vi "Config Mapping.vi"(8 "error in (no error)":errorcluster, 11 "HW InOut MAP in":T2) -> (0 "error out":errorcluster, 3 "HW InOut MAP out":T2)   [LabVIEW 2014, in "SeqLoop.lvlib"]
doc: "Configura el mapeo de entradas y salidas digitales."
uses:
  TypeDefs/HW InOut MAP.ctl
  SeqLoop.lvlib
panel:
  out "Array":T1(array[cluster])
  in  "IO Config":T3(tab)
  in  "Edit Map In":bool
  in  "I Config":i32(listbox)=-1 caption="Secuencia"
  in  "Add Map In":bool
  in  "Delete Map In":bool
  in  "Stop Map In":bool
  in  "Edit Map Out":bool
  in  "Out Config":i32(listbox)=-1 caption="Secuencia"
  in  "Add Map Out":bool
  in  "Delete Map Out":bool
  in  "Stop Map Out":bool
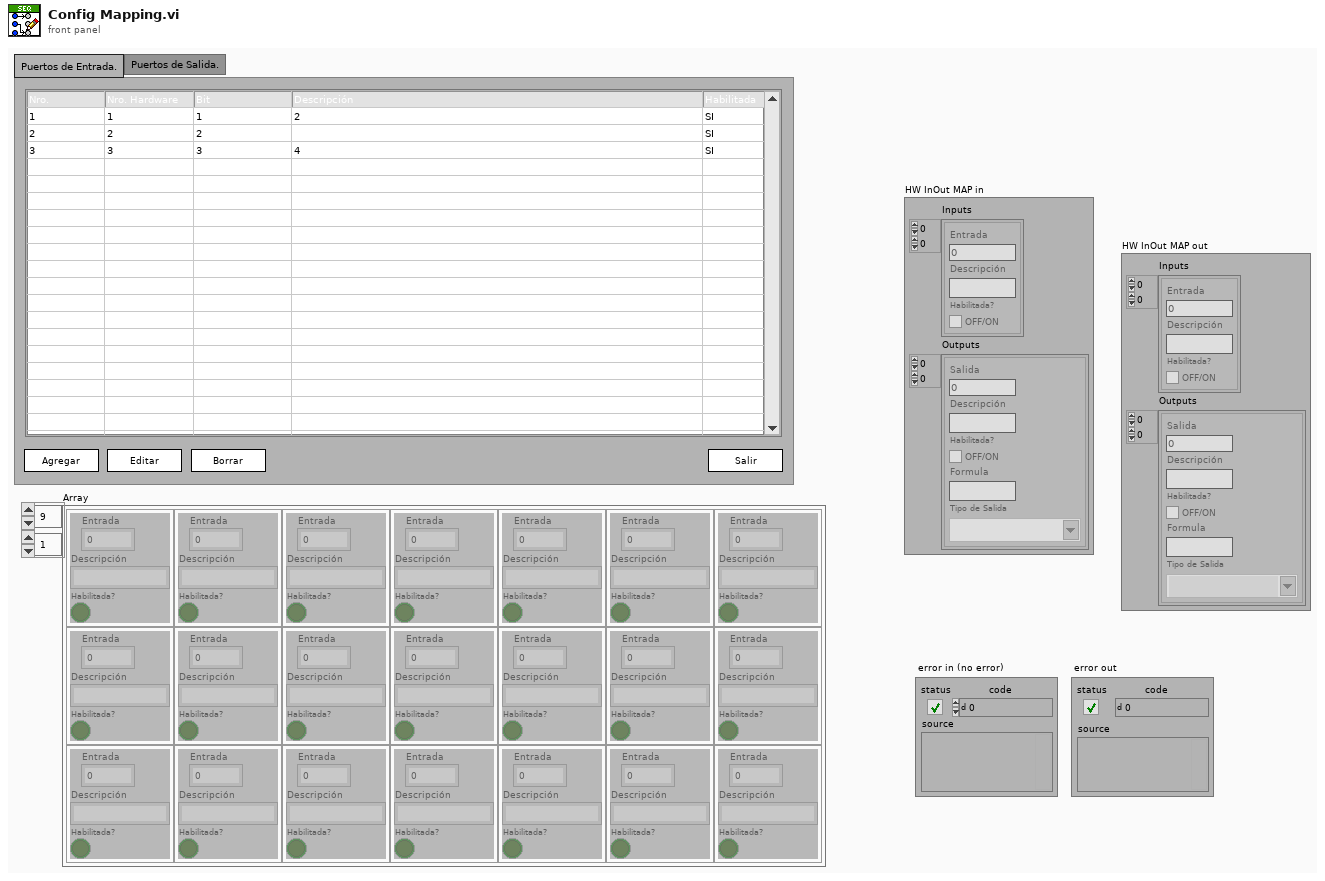
[diagram p1: front panel]
types:
  T1 = cluster{"Entrada":i32, "Descripción":string, "Habilitada?":bool}[][]
  T2 = typedef "SeqLoop.lvlib/HW InOut MAP.ctl" = cluster{"Inputs":cluster{"Entrada":i32, "Descripción":string, "Habilitada?":bool}[][], "Outputs":cluster{"Salida":i32, "Descripción":string, "Habilitada?":bool, "Formula":string, "Tipo de Salida":string}[][]}
  T3 = enum32{"Puertos de Entrada.", "Puertos de Salida."}
  T4 = cluster{"Entrada":i32, "Descripción":string, "Habilitada?":bool, "Formula":string, "Tipo de Salida":string}
  T5 = cluster{"Entrada":i32, "Descripción":string, "Habilitada?":bool}
  T6 = enum8{"Enabled", "Disabled", "Disabled and Grayed Out"}
  T7 = cluster{"Salida":i32, "Descripción":string, "Habilitada?":bool, "Formula":string, "Tipo de Salida":string}[][]
  T8 = cluster{"Entrada":i32, "Descripción":string, "Habilitada?":bool, "Formula":string, "Tipo de Salida":string}[][]
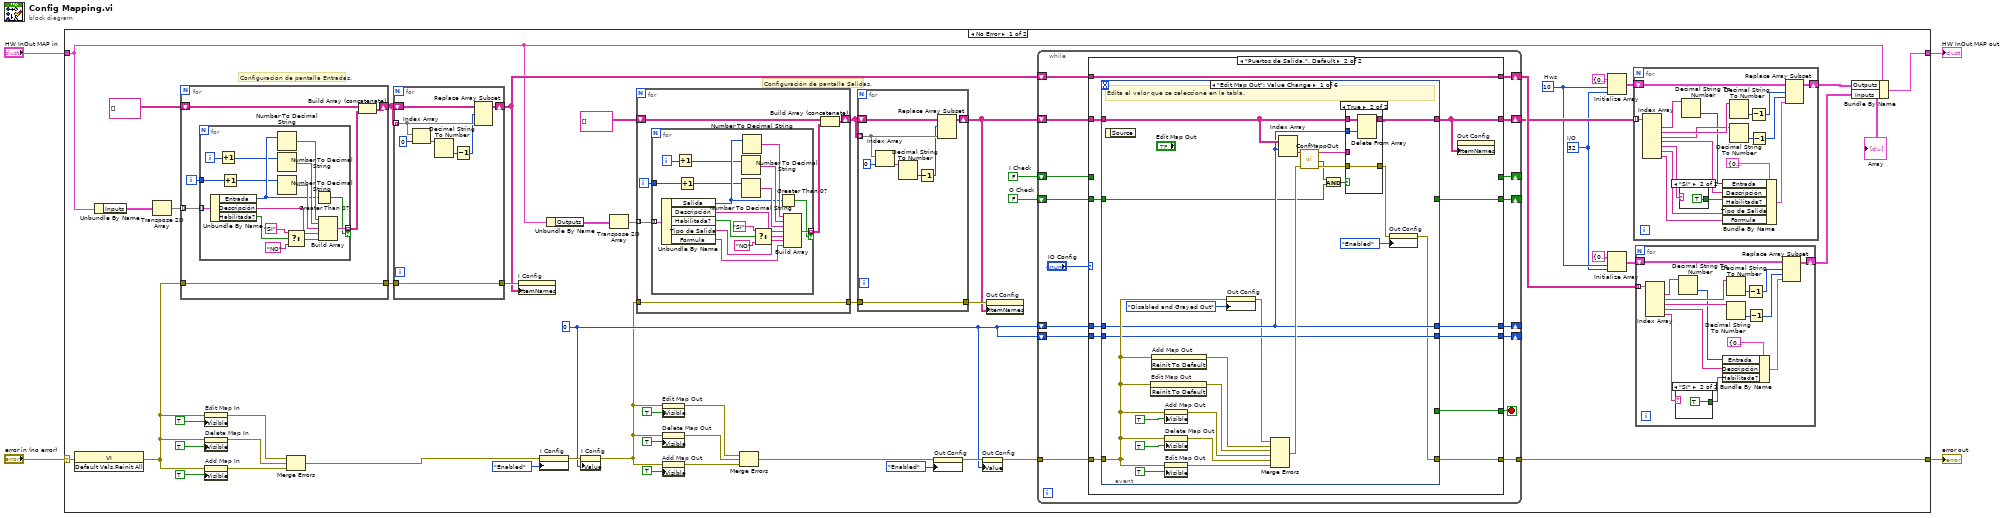
[diagram p0: block diagram]
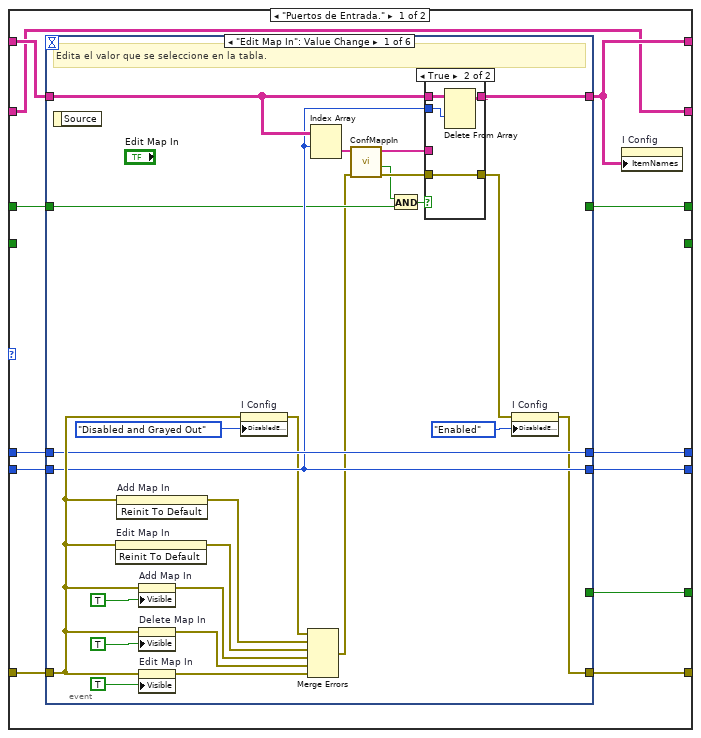
[diagram p4: hidden frame]
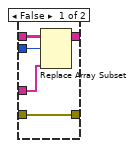
[diagram p5: hidden frame]
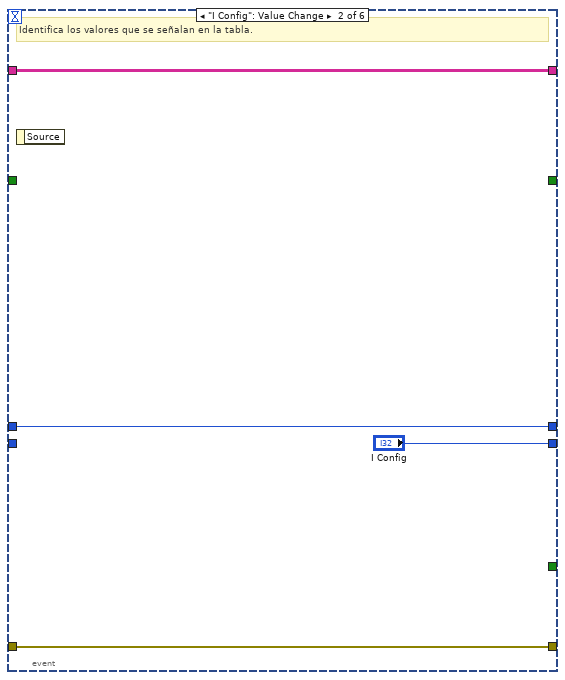
[diagram p6: hidden frame]
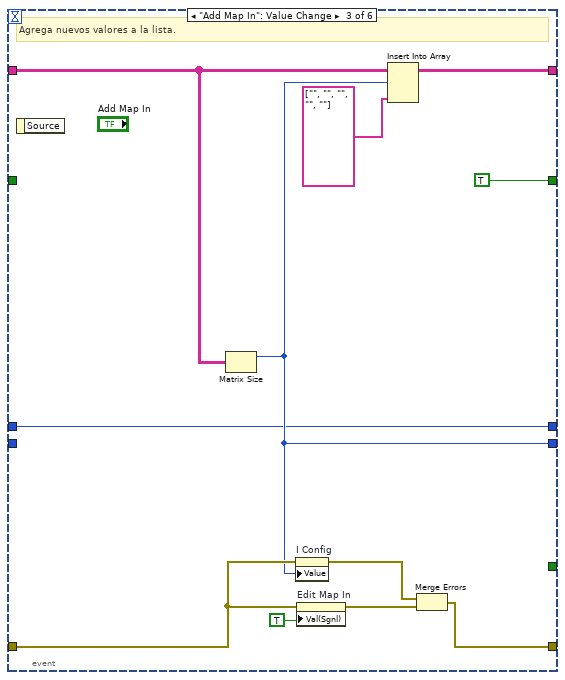
[diagram p7: hidden frame]
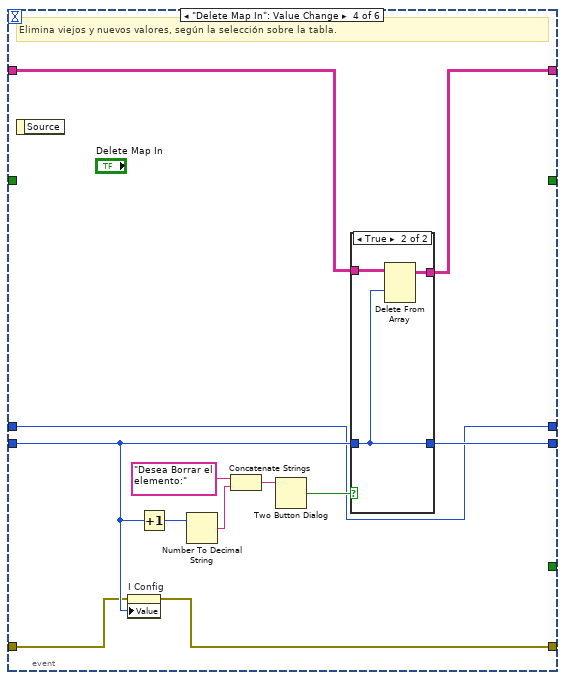
[diagram p8: hidden frame]
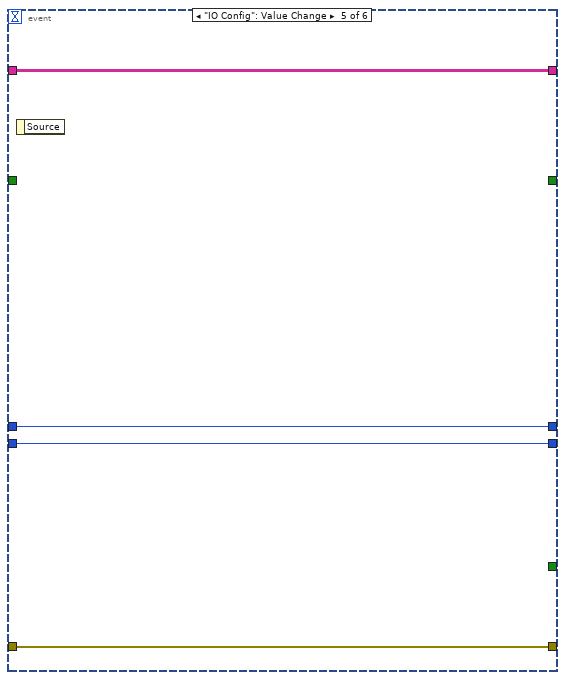
[diagram p10: hidden frame]
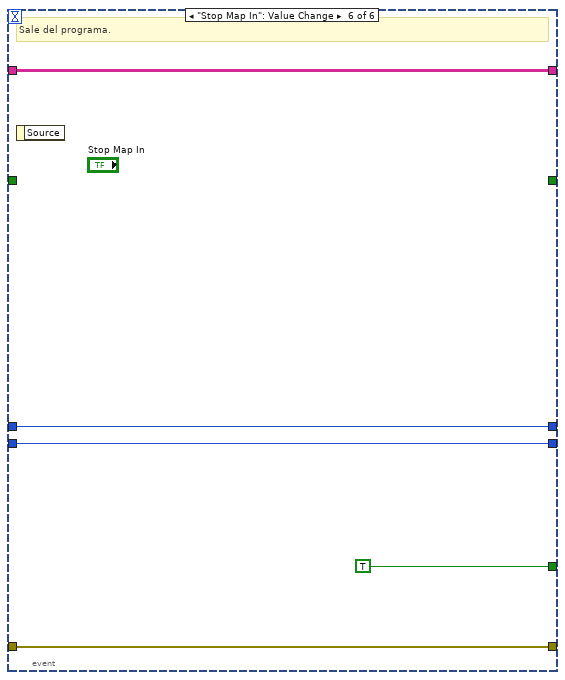
[diagram p11: hidden frame]
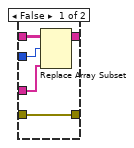
[diagram p12: hidden frame]
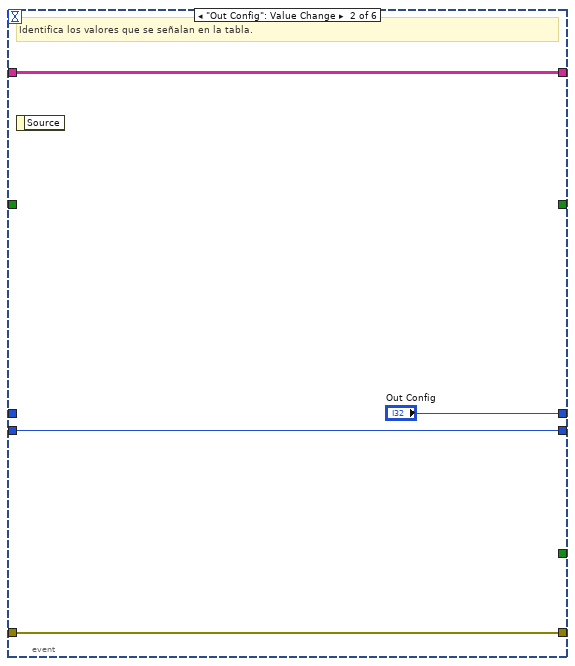
[diagram p13: hidden frame]
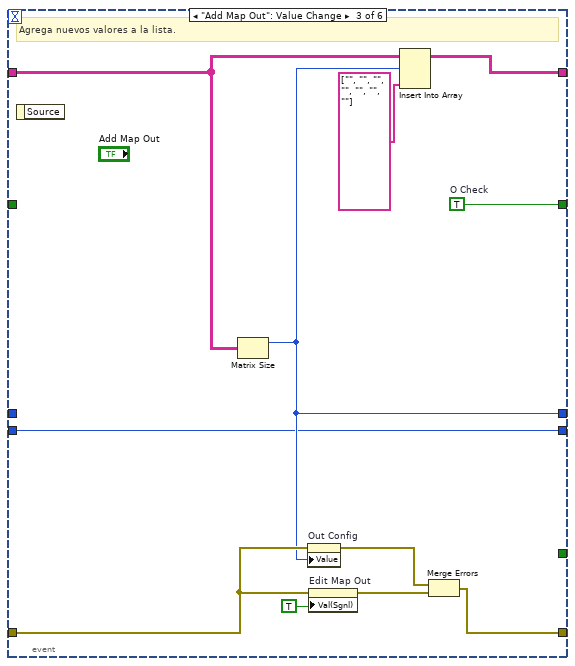
[diagram p14: hidden frame]
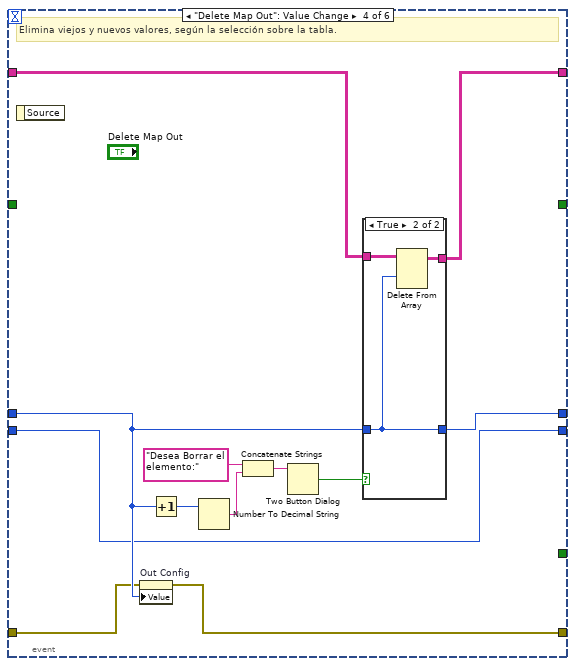
[diagram p15: hidden frame]
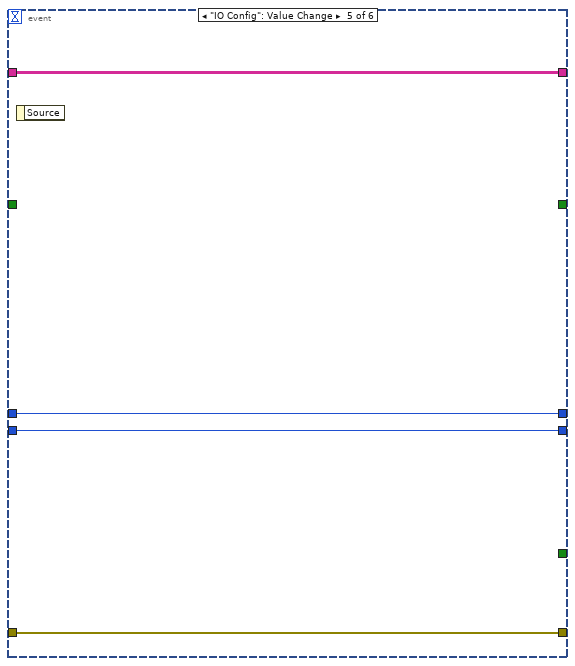
[diagram p17: hidden frame]
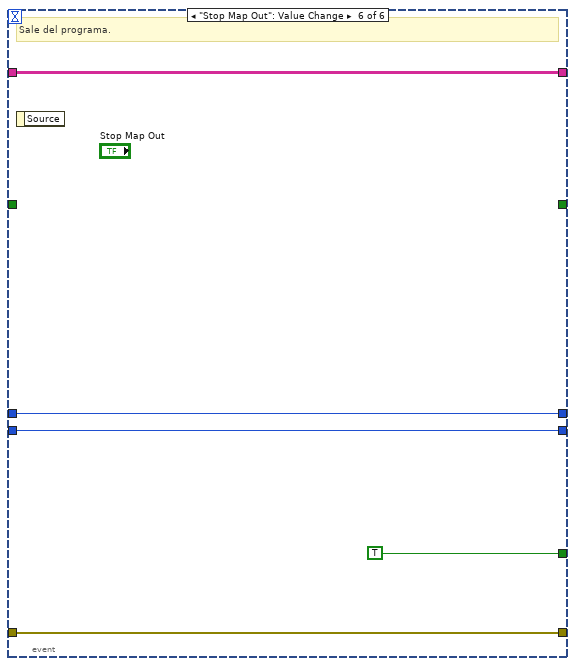
[diagram p18: hidden frame]
diagram:
  n1 = case shown="No Error" "error in (no error)" {
    selector: "error in (no error)" -> [w55 w346]
    tunnel: [w56 w346] -> w4
    tunnel: "HW InOut MAP in" -> [w19 w345]
    tunnel: [w34 w345] -> w1
    frame No Error {
      w5 = FALSE  # O Check
      w6 = FALSE  # I Check
      w11 = 32  # I/O
      w12 = 10  # Hws
      w36 = 0 ("disabled index (col)")
      # "Configuración de pantalla Entradas."
      # "Configuración de pantalla Salidas."
      n2 = invoke class="VI" method="Default Vals.Reinit All"(error in=w55) -> (error out=w22:errorcluster)  [unwired: 2 in, 2 out]
      n3 = Unbundle By Name(w19) -> ("Inputs"=w10:T1)
      n4 = Transpose 2D Array(2D array=w10) -> (transposed array=w9:T1)
      n5 = for {
        tunnel: w9 -> [w87] mode=indexing
        shift-right: [w83] -> w24
        shift-left: string[][] [] -> [w85]
        tunnel: w22 -> [w82]
        tunnel: [w82] -> w26
        i -> [w86]
        n6 = for {
          tunnel: w87 -> [w103] mode=indexing
          tunnel: w86 -> [w91]
          tunnel: [w98] -> w84 mode=indexing if=w92
          i -> [w89]
          n7 = Unbundle By Name(w103) -> ("Entrada"=w93:i32, "Descripción"=w94:string, "Habilitada?"=w102:bool)
          n8 = Increment(x=w89) -> (x+1=w88:i32)
          n9 = Increment(x=w91) -> (x+1=w90:i32)
          n10 = Number To Decimal String(number=w88) -> (decimal integer string=w97:string)  [unwired: 1 in]
          n11 = Number To Decimal String(number=w90) -> (decimal integer string=w96:string)  [unwired: 1 in]
          n12 = Number To Decimal String(number=w93) -> (decimal integer string=w99:string)  [unwired: 1 in]
          n13 = Select(t="SI" ("Descripción"), s=w102, f="NO" ("Descripción")) -> (s? t:f=w95:string)
          n14 = Greater Than 0?(x=w93) -> (x > 0?=w92:bool)
          n15 = Build Array(w99, w97, w96, w94, w95) -> (w98:string[])
        }
        n16 = Build Array (concatenate)(w85, w84) -> (w83:string[][])
      }
      n17 = property on="Edit Map In" class="Bool (strict)"(error in=w22, "Visible"=TRUE) -> (error out=w47:errorcluster)  [unwired: 1 in, 1 out]
      n18 = property on="Delete Map In" class="Bool"(error in=w22, "Visible"=TRUE) -> (error out=w49:errorcluster)  [unwired: 1 in, 1 out]
      n19 = property on="Add Map In" class="Bool (strict)"(error in=w22, "Visible"=TRUE) -> (error out=w51:errorcluster)  [unwired: 1 in, 1 out]
      n20 = Merge Errors(w47, w49, w51) -> (w53:errorcluster)
      n21 = for {
        tunnel: w24 -> [w79] mode=indexing
        shift-right: [w78] -> w21
        shift-left: w24 -> [w80]
        tunnel: [w74] -> w25
        tunnel: w26 -> [w74]
        n22 = Index Array(array=w79, index=0) -> (element=w77:string)
        n23 = Decimal String To Number(string=w77) -> (number=w76:i32)  [unwired: 2 in, 1 out]
        n24 = Decrement(x=w76) -> (x-1=w75:i32)
        n25 = Replace Array Subset(array=w80, new element=w79, index (row)=w75) -> (w78:string[][])  [unwired: 1 in]
      }
      n26 = property on="I Config" class="MCListbox (strict)"(error in=w25, "ItemNames"=w21) -> ()  [unwired: 1 in, 2 out]
      n27 = property on="I Config" class="MCListbox (strict)"(error in=w53, "DisabledEnum"=T6."Enabled" ("Disabled")) -> (error out=w54:errorcluster)  [unwired: 1 in, 1 out]
      n28 = Unbundle By Name(w19) -> ("Outputs"=w8:T7)
      n29 = property on="I Config" class="MCListbox (strict)"(error in=w54, "Value"=w36) -> (error out=w27:errorcluster)  [unwired: 1 in, 1 out]
      n30 = Transpose 2D Array(2D array=w8) -> (transposed array=w7:T7)
      n31 = for {
        tunnel: w7 -> [w117] mode=indexing
        shift-right: [w113] -> w30
        shift-left: string[][] [] -> [w115]
        tunnel: w27 -> [w112]
        tunnel: [w112] -> w32
        i -> [w116]
        n32 = for {
          tunnel: w117 -> [w135] mode=indexing
          tunnel: w116 -> [w123]
          tunnel: [w130] -> w114 mode=indexing if=w124
          i -> [w121]
          n33 = Unbundle By Name(w135) -> ("Salida"=w125:i32, "Descripción"=w126:string, "Habilitada?"=w134:bool, "Tipo de Salida"=w119:string, "Formula"=w118:string)
          n34 = Increment(x=w121) -> (x+1=w120:i32)
          n35 = Increment(x=w123) -> (x+1=w122:i32)
          n36 = Number To Decimal String(number=w120) -> (decimal integer string=w129:string)  [unwired: 1 in]
          n37 = Number To Decimal String(number=w122) -> (decimal integer string=w128:string)  [unwired: 1 in]
          n38 = Number To Decimal String(number=w125) -> (decimal integer string=w131:string)  [unwired: 1 in]
          n39 = Select(t="SI" ("Descripción"), s=w134, f="NO" ("Descripción")) -> (s? t:f=w127:string)
          n40 = Greater Than 0?(x=w125) -> (x > 0?=w124:bool)
          n41 = Build Array(w131, w129, w128, w126, w127, w119, w118) -> (w130:string[])
        }
        n42 = Build Array (concatenate)(w115, w114) -> (w113:string[][])
      }
      n43 = property on="Edit Map Out" class="Bool (strict)"(error in=w27, "Visible"=TRUE) -> (error out=w38:errorcluster)  [unwired: 1 in, 1 out]
      n44 = property on="Delete Map Out" class="Bool"(error in=w27, "Visible"=TRUE) -> (error out=w40:errorcluster)  [unwired: 1 in, 1 out]
      n45 = property on="Add Map Out" class="Bool (strict)"(error in=w27, "Visible"=TRUE) -> (error out=w42:errorcluster)  [unwired: 1 in, 1 out]
      n46 = Merge Errors(w38, w40, w42) -> (w44:errorcluster)
      n47 = for {
        tunnel: w30 -> [w109] mode=indexing
        shift-right: [w108] -> w28
        shift-left: w30 -> [w110]
        tunnel: [w104] -> w31
        tunnel: w32 -> [w104]
        n48 = Index Array(array=w109, index=0) -> (element=w107:string)
        n49 = Decimal String To Number(string=w107) -> (number=w106:i32)  [unwired: 2 in, 1 out]
        n50 = Decrement(x=w106) -> (x-1=w105:i32)
        n51 = Replace Array Subset(array=w110, new element=w109, index (row)=w105) -> (w108:string[][])  [unwired: 1 in]
      }
      n52 = property on="Out Config" class="MCListbox (strict)"(error in=w44, "DisabledEnum"=T6."Enabled" ("Disabled")) -> (error out=w45:errorcluster)  [unwired: 1 in, 1 out]
      n53 = property on="Out Config" class="MCListbox (strict)"(error in=w45, "Value"=w36) -> (error out=w33:errorcluster)  [unwired: 1 in, 1 out]
      n54 = property on="Out Config" class="MCListbox (strict)"(error in=w31, "ItemNames"=w28) -> ()  [unwired: 1 in, 2 out]
      n55 = while {
        tunnel: w33 -> [w169]
        tunnel: [w170] -> w56
        shift-right: [w166] -> _
        shift-left: w36 -> [w165]
        shift-right: [w164] -> _
        shift-left: w36 -> [w163]
        shift-right: [w162] -> w14
        shift-left: w28 -> [w161]
        shift-right: [w159] -> w17
        shift-left: w21 -> [w160]
        shift-right: [w157] -> _
        shift-left: w6 -> [w158]
        shift-right: [w155] -> _
        shift-left: w5 -> [w156]
        stop <- w167 stop-if-true
        n56 = case shown="\"Puertos de Salida.\", Default" "IO Config" {
          tunnel: [w182 w269] -> w170
          tunnel: w169 -> [w179 w264]
          tunnel: [w181 w268] -> w167
          tunnel: w165 -> [w176 w265]
          tunnel: [w180 w266] -> w166
          tunnel: [w178 w267] -> w164
          tunnel: w163 -> [w177 w263]
          tunnel: [w173 w262] -> w162
          tunnel: w161 -> [w173 w261]
          tunnel: w160 -> [w175 w260]
          tunnel: [w174 w260] -> w159
          tunnel: w158 -> [w172 _]
          tunnel: [w171 _] -> w157
          tunnel: w156 -> [_ w259]
          tunnel: [_ w258] -> w155
          frame "Puertos de Entrada." {
            n57 = event shown="[0] \"Edit Map In\": Value Change" {
              selector: _ -> [_ _ _ _ _ _]
              dyn-events: _ -> [_ _ _ _ _ _]
              timeout: _ -> [_ _ _ _ _ _]
              tunnel: w175 -> [w198 w220 w225 w241 w252 w256]
              tunnel: [w196 w220 w227 w240 w252 w256] -> w174
              tunnel: [w197 "I Config" w224 w242 w251 w255] -> w180
              tunnel: w176 -> [w197 _ _ w235 w251 w255]
              tunnel: w179 -> [w201 w218 w226 w234 w249 w257]
              tunnel: [w188 w218 w228 w233 w249 w257] -> w182
              tunnel: [_ _ _ _ _ TRUE ("Stop Med")] -> w181
              tunnel: w177 -> [w200 w217 w222 w232 w250 w253]
              tunnel: [w200 w217 w222 w232 w250 w253] -> w178
              tunnel: w172 -> [w195 _ _ _ _ _]
              tunnel: [_ _ TRUE _ _ _] -> w171
              event "Edit Map In": Value Change {
                # "Edita el valor que se seleccione en la tabla."
                n58 = event-data() -> ()  [unwired: 1 in, 1 out]
                n59 = invoke on="Edit Map In" class="Bool (strict)" method="Reinit To Default"(error in=w201) -> (error out=w193:errorcluster)  [unwired: 2 in, 2 out]
                n60 = invoke on="Add Map In" class="Bool (strict)" method="Reinit To Default"(error in=w201) -> (error out=w192:errorcluster)  [unwired: 2 in, 2 out]
                n61 = property on="Add Map In" class="Bool (strict)"(error in=w201, "Visible"=TRUE) -> (error out=w203:errorcluster)  [unwired: 1 in, 1 out]
                n62 = property on="Delete Map In" class="Bool"(error in=w201, "Visible"=TRUE) -> (error out=w205:errorcluster)  [unwired: 1 in, 1 out]
                n63 = property on="Edit Map In" class="Bool (strict)"(error in=w201, "Visible"=TRUE) -> (error out=w194:errorcluster)  [unwired: 1 in, 1 out]
                n64 = property on="I Config" class="MCListbox (strict)"(error in=w201, "DisabledEnum"=T6."Disabled and Grayed Out" ("Disabled")) -> (error out=w191:errorcluster)  [unwired: 1 in, 1 out]
                n65 = Merge Errors(w191, w192, w193, w203, w205, w194) -> (w184:errorcluster)
                n66 = Index Array(array=w198, index (row)=w197) -> (element=w187:string[])  [unwired: 1 in]
                n67 = call "ConfMappIn.vi"("error in (no error)"=w184, "ConfMap In"=w187) -> ("error out"=w185:errorcluster, "Discard?"=w183:bool, "ConfMap Out"=w186:string[])  [unwired: 7 in]
                n68 = And(x=w183, y=w195) -> (x .and. y?=w199:bool)
                n69 = case shown="True" w199 {
                  tunnel: w198 -> [w212 w215]
                  tunnel: w197 -> [w211 w213]
                  tunnel: w186 -> [w210 _]
                  tunnel: [w209 w214] -> w196
                  tunnel: w185 -> [w208 w216]
                  tunnel: [w208 w216] -> w189
                  frame False {
                    n70 = Replace Array Subset(array=w212, new element=w210, index (row)=w211) -> (w209:string[][])  [unwired: 1 in]
                  }
                  frame True {
                    n71 = Delete From Array(array=w215, index (row)=w213) -> (array with subset deleted=w214:string[][])  [unwired: 2 in, 1 out]
                  }
                }
                n72 = property on="I Config" class="MCListbox (strict)"(error in=w189, "DisabledEnum"=T6."Enabled" ("Disabled")) -> (error out=w188:errorcluster)  [unwired: 1 in, 1 out]
              }
              event "I Config": Value Change {
                # "Identifica los valores que se señalan en la tabla."
                n73 = event-data() -> ()  [unwired: 1 in, 1 out]
              }
              event "Add Map In": Value Change {
                # "Agrega nuevos valores a la lista."
                n74 = event-data() -> ()  [unwired: 1 in, 1 out]
                n75 = Matrix Size(0:w225) -> (1:w224:i32)  [unwired: 1 out]
                n76 = property on="I Config" class="MCListbox (strict)"(error in=w226, "Value"=w224) -> (error out=w229:errorcluster)  [unwired: 1 in, 1 out]
                n77 = property on="Edit Map In" class="Bool (strict)"(error in=w226, "Val(Sgnl)"=TRUE) -> (error out=w230:errorcluster)  [unwired: 1 in, 1 out]
                n78 = Insert Into Array(array=w225, index (row)=w224, new element=string[] ["", "", "", "", ""] ("new element/subarray")) -> (w227:string[][])  [unwired: 1 in]
                n79 = Merge Errors(w229, w230) -> (w228:errorcluster)
              }
              event "Delete Map In": Value Change {
                # "Elimina viejos y nuevos valores, según la selección sobre la tabla."
                n80 = event-data() -> ()  [unwired: 1 in, 1 out]
                n81 = property on="I Config" class="MCListbox (strict)"(error in=w234, "Value"=w235) -> (error out=w233:errorcluster)  [unwired: 1 in, 1 out]
                n82 = Increment(x=w235) -> (x+1=w236:i32)
                n83 = Number To Decimal String(number=w236) -> (decimal integer string=w238:string)  [unwired: 1 in]
                n84 = Concatenate Strings("Desea Borrar el elemento:" ("message"), w238) -> (w237:string)
                n85 = Two Button Dialog(message=w237) -> (T button?=w243:bool)  [unwired: 2 in]
                n86 = case shown="True" w243 {
                  tunnel: w241 -> [w244 w248]
                  tunnel: [w245 w246] -> w242
                  tunnel: w235 -> [w245 w246]
                  tunnel: [w244 w247] -> w240
                  frame False {
                  }
                  frame True {
                    n87 = Delete From Array(array=w248, index (row)=w246) -> (array with subset deleted=w247:string[][])  [unwired: 2 in, 1 out]
                  }
                }
              }
              event "IO Config": Value Change {
                n88 = event-data() -> ()  [unwired: 1 in, 1 out]
              }
              event "Stop Map In": Value Change {
                # "Sale del programa."
                n89 = event-data() -> ()  [unwired: 1 in, 1 out]
              }
            }
            n90 = property on="I Config" class="MCListbox (strict)"("ItemNames"=w174) -> ()  [unwired: 2 in, 2 out]
          }
          frame "Puertos de Salida.", Default {
            n91 = event shown="[0] \"Edit Map Out\": Value Change" {
              selector: _ -> [_ _ _ _ _ _]
              dyn-events: _ -> [_ _ _ _ _ _]
              timeout: _ -> [_ _ _ _ _ _]
              tunnel: w261 -> [w283 w307 w312 w328 w339 w343]
              tunnel: [w282 w307 w314 w327 w339 w343] -> w262
              tunnel: [w281 "Out Config" w311 w329 w338 w342] -> w267
              tunnel: w263 -> [w281 _ _ w322 w338 w342]
              tunnel: w264 -> [w288 w305 w313 w321 w336 w344]
              tunnel: [w270 w305 w315 w320 w336 w344] -> w269
              tunnel: [_ _ _ _ _ TRUE ("Stop Med")] -> w268
              tunnel: w265 -> [w285 w304 w309 w319 w337 w340]
              tunnel: [w285 w304 w309 w319 w337 w340] -> w266
              tunnel: w259 -> [w278 _ _ _ _ _]
              tunnel: [_ _ w308 _ _ _] -> w258
              event "Edit Map Out": Value Change {
                # "Edita el valor que se seleccione en la tabla."
                n92 = event-data() -> ()  [unwired: 1 in, 1 out]
                n93 = invoke on="Edit Map Out" class="Bool (strict)" method="Reinit To Default"(error in=w288) -> (error out=w276:errorcluster)  [unwired: 2 in, 2 out]
                n94 = invoke on="Add Map Out" class="Bool (strict)" method="Reinit To Default"(error in=w288) -> (error out=w275:errorcluster)  [unwired: 2 in, 2 out]
                n95 = property on="Add Map Out" class="Bool (strict)"(error in=w288, "Visible"=TRUE) -> (error out=w290:errorcluster)  [unwired: 1 in, 1 out]
                n96 = property on="Delete Map Out" class="Bool"(error in=w288, "Visible"=TRUE) -> (error out=w292:errorcluster)  [unwired: 1 in, 1 out]
                n97 = property on="Edit Map Out" class="Bool (strict)"(error in=w288, "Visible"=TRUE) -> (error out=w277:errorcluster)  [unwired: 1 in, 1 out]
                n98 = property on="Out Config" class="MCListbox (strict)"(error in=w288, "DisabledEnum"=T6."Disabled and Grayed Out" ("Disabled")) -> (error out=w274:errorcluster)  [unwired: 1 in, 1 out]
                n99 = Merge Errors(w274, w275, w276, w290, w292, w277) -> (w286:errorcluster)
                n100 = Index Array(array=w283, index (row)=w281) -> (element=w287:string[])  [unwired: 1 in]
                n101 = call "ConfMappOut.vi"("error in (no error)"=w286, "ConfMapOut In"=w287) -> ("error out"=w279:errorcluster, "Discard?"=w273:bool, "ConfMapOut Out"=w280:string[])  [unwired: 7 in]
                n102 = And(x=w273, y=w278) -> (x .and. y?=w284:bool)
                n103 = case shown="True" w284 {
                  tunnel: w283 -> [w299 w302]
                  tunnel: w281 -> [w298 w300]
                  tunnel: w280 -> [w297 _]
                  tunnel: [w296 w301] -> w282
                  tunnel: w279 -> [w295 w303]
                  tunnel: [w295 w303] -> w271
                  frame False {
                    n104 = Replace Array Subset(array=w299, new element=w297, index (row)=w298) -> (w296:string[][])  [unwired: 1 in]
                  }
                  frame True {
                    n105 = Delete From Array(array=w302, index (row)=w300) -> (array with subset deleted=w301:string[][])  [unwired: 2 in, 1 out]
                  }
                }
                n106 = property on="Out Config" class="MCListbox (strict)"(error in=w271, "DisabledEnum"=T6."Enabled" ("Disabled")) -> (error out=w270:errorcluster)  [unwired: 1 in, 1 out]
              }
              event "Out Config": Value Change {
                # "Identifica los valores que se señalan en la tabla."
                n107 = event-data() -> ()  [unwired: 1 in, 1 out]
              }
              event "Add Map Out": Value Change {
                w308 = TRUE  # O Check
                # "Agrega nuevos valores a la lista."
                n108 = event-data() -> ()  [unwired: 1 in, 1 out]
                n109 = Matrix Size(0:w312) -> (1:w311:i32)  [unwired: 1 out]
                n110 = property on="Out Config" class="MCListbox (strict)"(error in=w313, "Value"=w311) -> (error out=w316:errorcluster)  [unwired: 1 in, 1 out]
                n111 = property on="Edit Map Out" class="Bool (strict)"(error in=w313, "Val(Sgnl)"=TRUE) -> (error out=w317:errorcluster)  [unwired: 1 in, 1 out]
                n112 = Insert Into Array(array=w312, index (row)=w311, new element=string[] ["", "", "", "", "", "", ""] ("new element/subarray")) -> (w314:string[][])  [unwired: 1 in]
                n113 = Merge Errors(w316, w317) -> (w315:errorcluster)
              }
              event "Delete Map Out": Value Change {
                # "Elimina viejos y nuevos valores, según la selección sobre la tabla."
                n114 = event-data() -> ()  [unwired: 1 in, 1 out]
                n115 = property on="Out Config" class="MCListbox (strict)"(error in=w321, "Value"=w322) -> (error out=w320:errorcluster)  [unwired: 1 in, 1 out]
                n116 = Increment(x=w322) -> (x+1=w323:i32)
                n117 = Number To Decimal String(number=w323) -> (decimal integer string=w325:string)  [unwired: 1 in]
                n118 = Concatenate Strings("Desea Borrar el elemento:" ("message"), w325) -> (w324:string)
                n119 = Two Button Dialog(message=w324) -> (T button?=w330:bool)  [unwired: 2 in]
                n120 = case shown="True" w330 {
                  tunnel: w328 -> [w331 w335]
                  tunnel: [w332 w333] -> w329
                  tunnel: w322 -> [w332 w333]
                  tunnel: [w331 w334] -> w327
                  frame False {
                  }
                  frame True {
                    n121 = Delete From Array(array=w335, index (row)=w333) -> (array with subset deleted=w334:string[][])  [unwired: 2 in, 1 out]
                  }
                }
              }
              event "IO Config": Value Change {
                n122 = event-data() -> ()  [unwired: 1 in, 1 out]
              }
              event "Stop Map Out": Value Change {
                # "Sale del programa."
                n123 = event-data() -> ()  [unwired: 1 in, 1 out]
              }
            }
            n124 = property on="Out Config" class="MCListbox (strict)"("ItemNames"=w262) -> ()  [unwired: 2 in, 2 out]
          }
        }
      }
      n125 = Initialize Array(T4 {"Entrada"=0, "Descripción"="", "Habilitada?"=FALSE, "Formula"="", "Tipo de Salida"=""} ("Cluster"), w12, w11) -> (w15:T8)
      n126 = Initialize Array(T5 {"Entrada"=0, "Descripción"="", "Habilitada?"=FALSE} ("Cluster"), w12, w11) -> (w16:T1)
      n127 = for {
        tunnel: w14 -> [w153] mode=indexing
        shift-right: [w140] -> w35
        shift-left: w15 -> [w139]
        n128 = Index Array(array=w153) -> (element #1=w147:string, element #2=w152:string, element #3=w151:string, element #4=w148:string, element #5=w150:string, element #6=w137:string, element #7=w136:string)  [unwired: 7 in]
        n129 = case shown="\"SI\"" w150 {
          tunnel: [_ TRUE] -> w149
          frame "NO", Default {
          }
          frame "SI" {
          }
        }
        n130 = Decimal String To Number(string=w147) -> (number=w146:i32)  [unwired: 2 in, 1 out]
        n131 = Bundle By Name(cluster=T4 {"Entrada"=0, "Descripción"="", "Habilitada?"=FALSE, "Formula"="", "Tipo de Salida"=""} ("Cluster"), "Entrada"=w146, "Descripción"=w148, "Habilitada?"=w149, "Tipo de Salida"=w137, "Formula"=w136) -> (w145:T4)
        n132 = Decimal String To Number(string=w152) -> (number=w143:i32)  [unwired: 2 in, 1 out]
        n133 = Decimal String To Number(string=w151) -> (number=w142:i32)  [unwired: 2 in, 1 out]
        n134 = Decrement(x=w143) -> (x-1=w144:i32)
        n135 = Decrement(x=w142) -> (x-1=w141:i32)
        n136 = Replace Array Subset(array=w139, new element=w145, index (row)=w144, index (col)=w141) -> (w140:T8)
      }
      n137 = for {
        tunnel: w17 -> [w72] mode=indexing
        shift-right: [w58] -> w20
        shift-left: w16 -> [w57]
        n138 = Index Array(array=w72) -> (element #1=w65:string, element #2=w70:string, element #3=w69:string, element #4=w66:string, element #5=w68:string)  [unwired: 5 in]
        n139 = case shown="\"SI\"" w68 {
          tunnel: [_ TRUE] -> w67
          frame "NO", Default {
          }
          frame "SI" {
          }
        }
        n140 = Decimal String To Number(string=w65) -> (number=w64:i32)  [unwired: 2 in, 1 out]
        n141 = Bundle By Name(cluster=T5 {"Entrada"=0, "Descripción"="", "Habilitada?"=FALSE} ("Cluster"), "Entrada"=w64, "Descripción"=w66, "Habilitada?"=w67) -> (w63:T5)
        n142 = Decimal String To Number(string=w70) -> (number=w61:i32)  [unwired: 2 in, 1 out]
        n143 = Decimal String To Number(string=w69) -> (number=w60:i32)  [unwired: 2 in, 1 out]
        n144 = Decrement(x=w61) -> (x-1=w62:i32)
        n145 = Decrement(x=w60) -> (x-1=w59:i32)
        n146 = Replace Array Subset(array=w57, new element=w63, index (row)=w62, index (col)=w59) -> (w58:T1)
      }
      "Array" <- w20
      n147 = Bundle By Name(cluster=w19, "Outputs"=w35, "Inputs"=w20) -> (w34:T2)
    }
    frame Error {
    }
  }
  "error out" <- w4
  "HW InOut MAP out" <- w1
